vi "Main.vi"(8 "error in":errorcluster, 11 "gRPC Client in":refnum<class "gRPC Client.lvclass">) -> (0 "error out":errorcluster, 3 "gRPC Client out":refnum<class "gRPC Client.lvclass">)   [LabVIEW 2019, in "gRPC Client (template.proto).lvlib" / "gRPC Client.lvclass"]
doc: "The <b>Queued Message Handler</b> of the Worker that owns this VI."
uses:
  gRPC Client.lvclass
  C:/Program Files (x86)/National Instruments/LabVIEW 2019/vi.lib/addons/_Workers/Library/Classes/Worker/Worker.lvclass
  Initialization Data.ctl
  Response Cases.ctl
  <vilib>/addons/_Workers/Library/Case Label.ctl
  gRPC Client.lvclass/gRPC Client.ctl
  rwr_Create gRPC Client.ctl
  rwr_Create gRPC Client Reply.ctl
  rwr_Destroy gRPC Client.ctl
  rwr_Destroy gRPC Client Reply.ctl
  rqp_Msg_ToServer_1.ctl
  Generated_client/RPC Messages/w4lvgrpc_Msg_ToServer_1.ctl
  Generated_client/RPC Messages/w4lvgrpc_ToServer.ctl
  Generated_client/RPC Messages/w4lvgrpc_ToServer_payload/w4lvgrpc_ToServer_payload.lvclass
  Generated_client/RPC Messages/w4lvgrpc_ToServer_payload/w4lvgrpc_ToServer_payload.lvclass/w4lvgrpc_ToServer_payload.ctl
  rqp_Msg_ToServer_2.ctl
  Generated_client/RPC Messages/w4lvgrpc_Msg_ToServer_2.ctl
  rqp_Msg_ToServer_3.ctl
  Generated_client/RPC Messages/w4lvgrpc_Msg_ToServer_3.ctl
  rqp_Msg_ToServer_4.ctl
  Generated_client/RPC Messages/w4lvgrpc_Msg_ToServer_4.ctl
  rqp_Msg_ToServer_5.ctl
  Generated_client/RPC Messages/w4lvgrpc_Msg_ToServer_5.ctl
  rqp_Msg_ToServer_6.ctl
  Generated_client/RPC Messages/w4lvgrpc_Msg_ToServer_6.ctl
  rqp_Msg_ToServer_7.ctl
  Generated_client/RPC Messages/w4lvgrpc_Msg_ToServer_7.ctl
  rqp_Msg_ToServer_8.ctl
  Generated_client/RPC Messages/w4lvgrpc_Msg_ToServer_8.ctl
  rqp_Msg_ToServer_9.ctl
  Generated_client/RPC Messages/w4lvgrpc_Msg_ToServer_9.ctl
  Generated_client/RPC Messages/w4lvgrpc_ToClient_payload/w4lvgrpc_ToClient_payload.lvclass/w4lvgrpc_ToClient_payload.ctl
  rsp_Msg_ToClient_1.ctl
  Generated_client/RPC Messages/w4lvgrpc_Msg_ToClient_1.ctl
  rsp_Msg_ToClient_2.ctl
  Generated_client/RPC Messages/w4lvgrpc_Msg_ToClient_2.ctl
  rsp_Msg_ToClient_3.ctl
  Generated_client/RPC Messages/w4lvgrpc_Msg_ToClient_3.ctl
  rsp_Msg_ToClient_4.ctl
  Generated_client/RPC Messages/w4lvgrpc_Msg_ToClient_4.ctl
  rsp_Msg_ToClient_5.ctl
  Generated_client/RPC Messages/w4lvgrpc_Msg_ToClient_5.ctl
  rsp_Msg_ToClient_6.ctl
  Generated_client/RPC Messages/w4lvgrpc_Msg_ToClient_6.ctl
  rsp_Msg_ToClient_7.ctl
  Generated_client/RPC Messages/w4lvgrpc_Msg_ToClient_7.ctl
  rsp_Msg_ToClient_8.ctl
  Generated_client/RPC Messages/w4lvgrpc_Msg_ToClient_8.ctl
  rsp_Msg_ToClient_9.ctl
  Generated_client/RPC Messages/w4lvgrpc_Msg_ToClient_9.ctl
  <vilib>/Utility/error.llb/Error Cluster From Error Code.vi
  <vilib>/ErrorRing/Error Ring.xnode
  <vilib>/addons/_Workers/Library/Workers.lvlib
  gRPC Read/gRPC Read.lvclass
  Generated_client/Generated_client.lvlib
  Generated_client/RPC Messages/w4lvgrpc_ToClient_payload/w4lvgrpc_ToClient_payload.lvclass
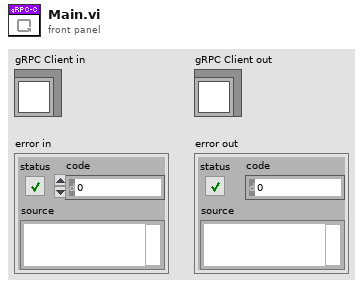
[diagram p1: front panel]
types:
  T1 = typedef "gRPC Client (template.proto).lvlib/gRPC Client.lvclass/Initialization Data.ctl" = cluster{"Response Cases":T2}
  T2 = typedef "gRPC Client (template.proto).lvlib/gRPC Client.lvclass/Response Cases.ctl" = cluster{"Connection Notify":T3, "Client Error":T3, "Msg_ToClient_1":T3, "Msg_ToClient_2":T3, "Msg_ToClient_3":T3, "Msg_ToClient_4":T3, "Msg_ToClient_5":T3, "Msg_ToClient_6":T3, "Msg_ToClient_7":T3, "Msg_ToClient_8":T3, "Msg_ToClient_9":T3}
  T3 = typedef "Workers.lvlib/Case Label.ctl" = string
  T4 = typedef "gRPC Client (template.proto).lvlib/gRPC Client.lvclass/rwr_Create gRPC Client Reply.ctl" = cluster{"Placeholder":string}
  T5 = typedef "gRPC Client (template.proto).lvlib/gRPC Client.lvclass/rwr_Create gRPC Client.ctl" = cluster{"Server Address":string, "Certificate Path":string}
  T6 = typedef "gRPC Client (template.proto).lvlib/gRPC Client.lvclass/rwr_Destroy gRPC Client Reply.ctl" = cluster{"String":string}
  T7 = typedef "gRPC Client (template.proto).lvlib/gRPC Client.lvclass/rwr_Destroy gRPC Client.ctl" = cluster{"Placeholder":string}
  T8 = typedef "Generated_client.lvlib/w4lvgrpc_ToServer.ctl" = cluster{"w4lvgrpc_ToServer_payload":refnum<class "w4lvgrpc_ToServer_payload.lvclass">}
  T9 = typedef "gRPC Client (template.proto).lvlib/gRPC Client.lvclass/rqp_Msg_ToServer_1.ctl" = cluster{"w4lvgrpc_Msg_ToServer_1":T10}
  T10 = typedef "Generated_client.lvlib/w4lvgrpc_Msg_ToServer_1.ctl" = cluster{"placeholder":string}
  T11 = typedef "gRPC Client (template.proto).lvlib/gRPC Client.lvclass/rqp_Msg_ToServer_2.ctl" = cluster{"w4lvgrpc_Msg_ToServer_2":T12}
  T12 = typedef "Generated_client.lvlib/w4lvgrpc_Msg_ToServer_2.ctl" = cluster{"placeholder":string}
  T13 = typedef "gRPC Client (template.proto).lvlib/gRPC Client.lvclass/rqp_Msg_ToServer_3.ctl" = cluster{"w4lvgrpc_Msg_ToServer_3":T14}
  T14 = typedef "Generated_client.lvlib/w4lvgrpc_Msg_ToServer_3.ctl" = cluster{"placeholder":string}
  T15 = typedef "gRPC Client (template.proto).lvlib/gRPC Client.lvclass/rqp_Msg_ToServer_4.ctl" = cluster{"w4lvgrpc_Msg_ToServer_4":T16}
  T16 = typedef "Generated_client.lvlib/w4lvgrpc_Msg_ToServer_4.ctl" = cluster{"placeholder":string}
  T17 = typedef "gRPC Client (template.proto).lvlib/gRPC Client.lvclass/rqp_Msg_ToServer_5.ctl" = cluster{"w4lvgrpc_Msg_ToServer_5":T18}
  T18 = typedef "Generated_client.lvlib/w4lvgrpc_Msg_ToServer_5.ctl" = cluster{"placeholder":string}
  T19 = typedef "gRPC Client (template.proto).lvlib/gRPC Client.lvclass/rqp_Msg_ToServer_6.ctl" = cluster{"w4lvgrpc_Msg_ToServer_6":T20}
  T20 = typedef "Generated_client.lvlib/w4lvgrpc_Msg_ToServer_6.ctl" = cluster{"placeholder":string}
  T21 = typedef "gRPC Client (template.proto).lvlib/gRPC Client.lvclass/rqp_Msg_ToServer_7.ctl" = cluster{"w4lvgrpc_Msg_ToServer_7":T22}
  T22 = typedef "Generated_client.lvlib/w4lvgrpc_Msg_ToServer_7.ctl" = cluster{"placeholder":string}
  T23 = typedef "gRPC Client (template.proto).lvlib/gRPC Client.lvclass/rqp_Msg_ToServer_8.ctl" = cluster{"w4lvgrpc_Msg_ToServer_8":T24}
  T24 = typedef "Generated_client.lvlib/w4lvgrpc_Msg_ToServer_8.ctl" = cluster{"placeholder":string}
  T25 = typedef "gRPC Client (template.proto).lvlib/gRPC Client.lvclass/rqp_Msg_ToServer_9.ctl" = cluster{"w4lvgrpc_Msg_ToServer_9":T26}
  T26 = typedef "Generated_client.lvlib/w4lvgrpc_Msg_ToServer_9.ctl" = cluster{"placeholder":string}
  T27 = typedef "gRPC Client (template.proto).lvlib/gRPC Client.lvclass/rsp_Msg_ToClient_1.ctl" = cluster{"w4lvgrpc_Msg_ToClient_1":T28}
  T28 = typedef "Generated_client.lvlib/w4lvgrpc_Msg_ToClient_1.ctl" = cluster{"placeholder":string}
  T29 = typedef "gRPC Client (template.proto).lvlib/gRPC Client.lvclass/rsp_Msg_ToClient_2.ctl" = cluster{"w4lvgrpc_Msg_ToClient_2":T30}
  T30 = typedef "Generated_client.lvlib/w4lvgrpc_Msg_ToClient_2.ctl" = cluster{"placeholder":string}
  T31 = typedef "gRPC Client (template.proto).lvlib/gRPC Client.lvclass/rsp_Msg_ToClient_3.ctl" = cluster{"w4lvgrpc_Msg_ToClient_3":T32}
  T32 = typedef "Generated_client.lvlib/w4lvgrpc_Msg_ToClient_3.ctl" = cluster{"placeholder":string}
  T33 = typedef "gRPC Client (template.proto).lvlib/gRPC Client.lvclass/rsp_Msg_ToClient_4.ctl" = cluster{"w4lvgrpc_Msg_ToClient_4":T34}
  T34 = typedef "Generated_client.lvlib/w4lvgrpc_Msg_ToClient_4.ctl" = cluster{"placeholder":string}
  T35 = typedef "gRPC Client (template.proto).lvlib/gRPC Client.lvclass/rsp_Msg_ToClient_5.ctl" = cluster{"w4lvgrpc_Msg_ToClient_5":T36}
  T36 = typedef "Generated_client.lvlib/w4lvgrpc_Msg_ToClient_5.ctl" = cluster{"placeholder":string}
  T37 = typedef "gRPC Client (template.proto).lvlib/gRPC Client.lvclass/rsp_Msg_ToClient_6.ctl" = cluster{"w4lvgrpc_Msg_ToClient_6":T38}
  T38 = typedef "Generated_client.lvlib/w4lvgrpc_Msg_ToClient_6.ctl" = cluster{"placeholder":string}
  T39 = typedef "gRPC Client (template.proto).lvlib/gRPC Client.lvclass/rsp_Msg_ToClient_7.ctl" = cluster{"w4lvgrpc_Msg_ToClient_7":T40}
  T40 = typedef "Generated_client.lvlib/w4lvgrpc_Msg_ToClient_7.ctl" = cluster{"placeholder":string}
  T41 = typedef "gRPC Client (template.proto).lvlib/gRPC Client.lvclass/rsp_Msg_ToClient_8.ctl" = cluster{"w4lvgrpc_Msg_ToClient_8":T42}
  T42 = typedef "Generated_client.lvlib/w4lvgrpc_Msg_ToClient_8.ctl" = cluster{"placeholder":string}
  T43 = typedef "gRPC Client (template.proto).lvlib/gRPC Client.lvclass/rsp_Msg_ToClient_9.ctl" = cluster{"w4lvgrpc_Msg_ToClient_9":T44}
  T44 = typedef "Generated_client.lvlib/w4lvgrpc_Msg_ToClient_9.ctl" = cluster{"placeholder":string}
  T45 = typedef "grpc-lvsupport-release.lvlib/grpcId.ctl" = u64
  T46 = typedef "gRPC Client (template.proto).lvlib/gRPC Read.lvclass/rsp_Receive Incoming gRPC Data.ctl" = refnum<class "w4lvgrpc_ToClient_payload.lvclass">
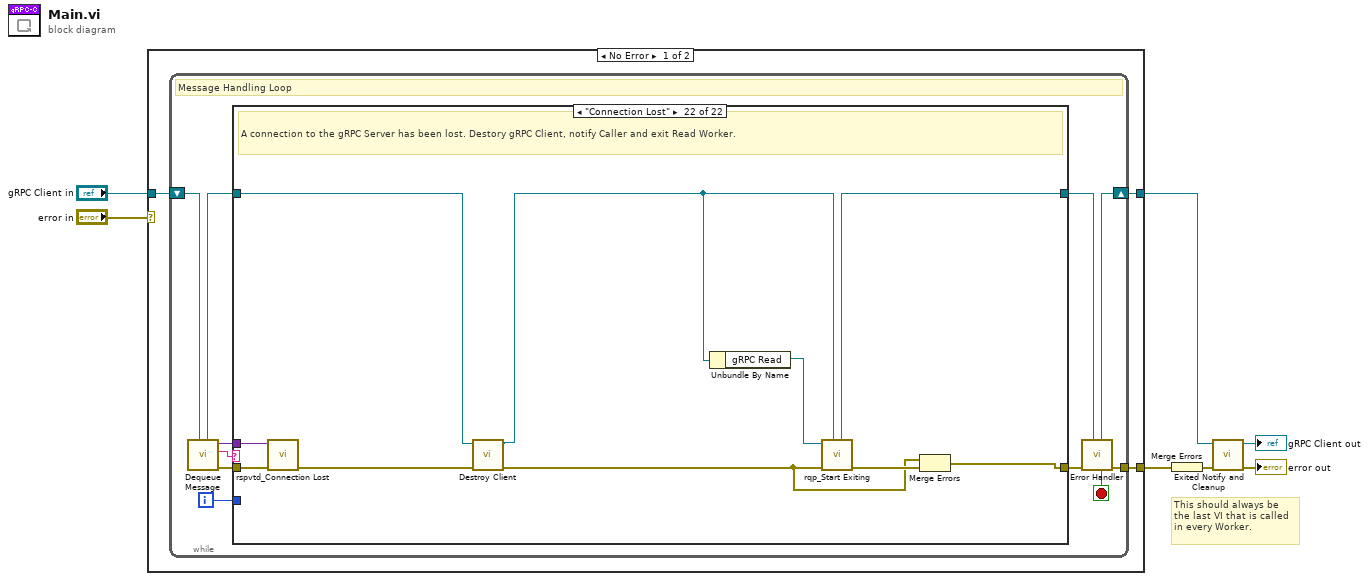
[diagram p0: block diagram]
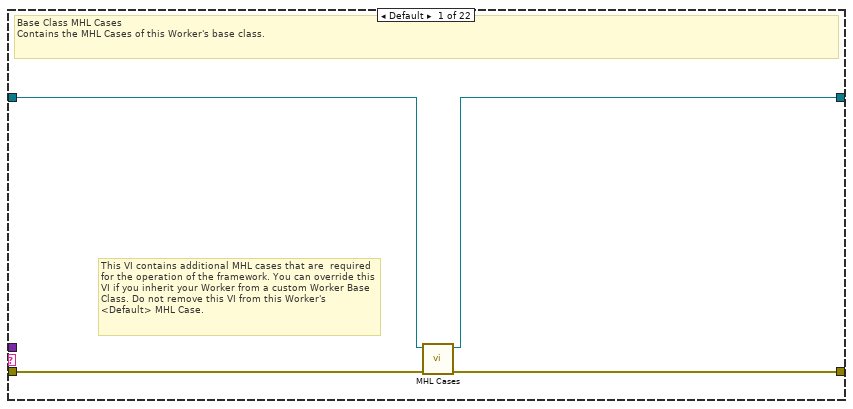
[diagram p2: hidden frame]
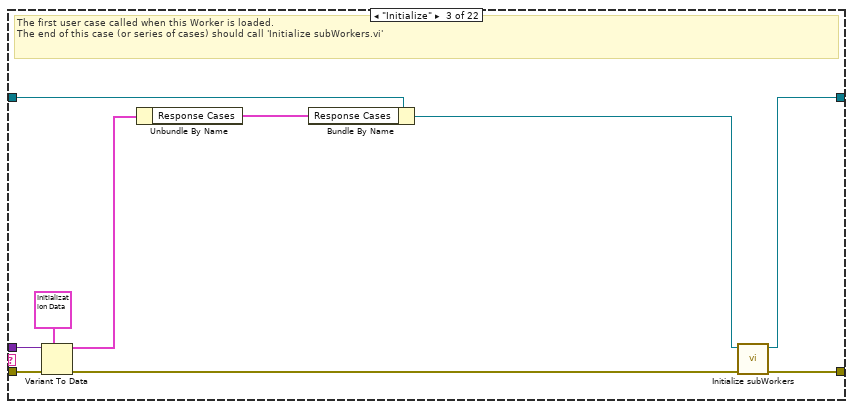
[diagram p4: hidden frame]
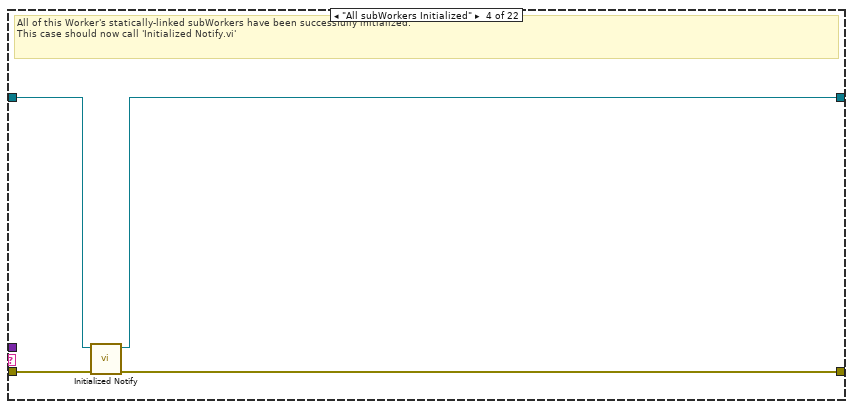
[diagram p5: hidden frame]
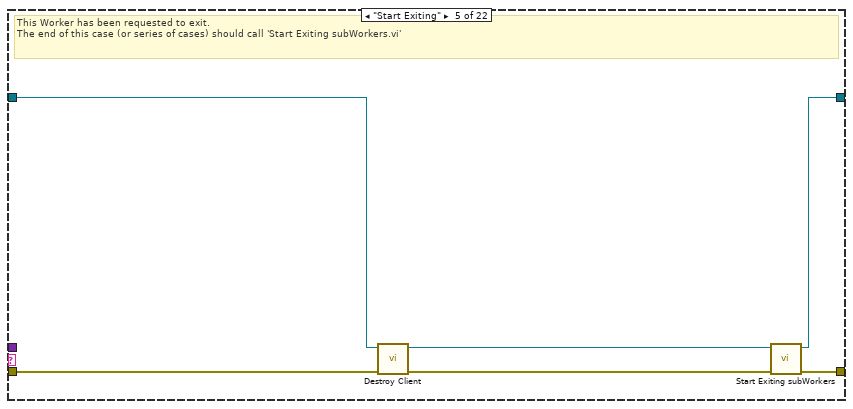
[diagram p6: hidden frame]
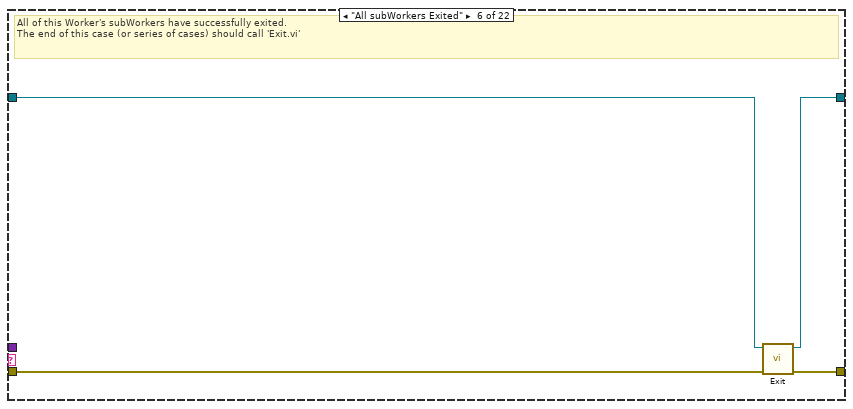
[diagram p7: hidden frame]
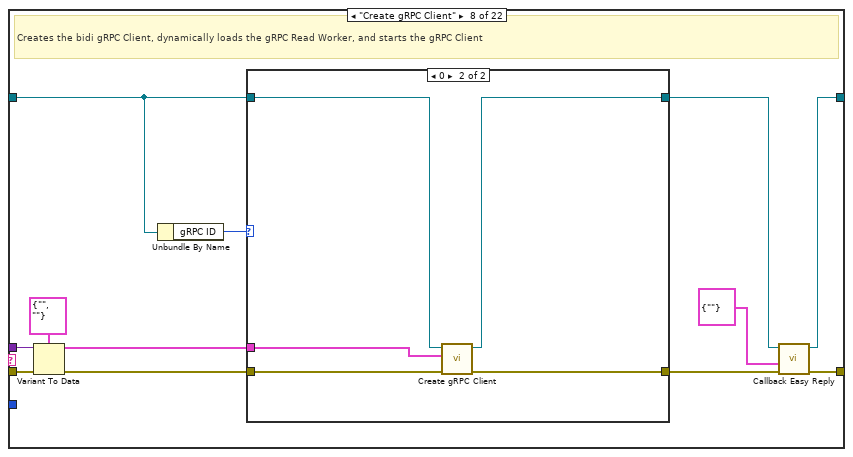
[diagram p9: hidden frame]
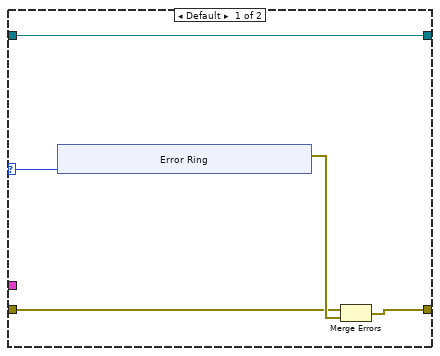
[diagram p10: hidden frame]
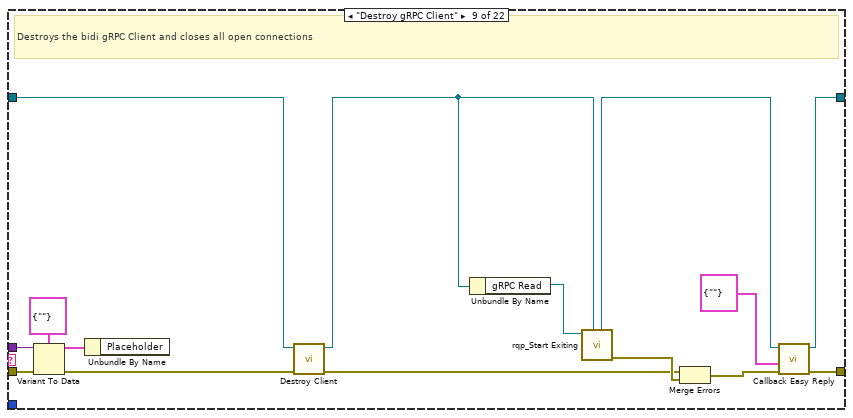
[diagram p11: hidden frame]
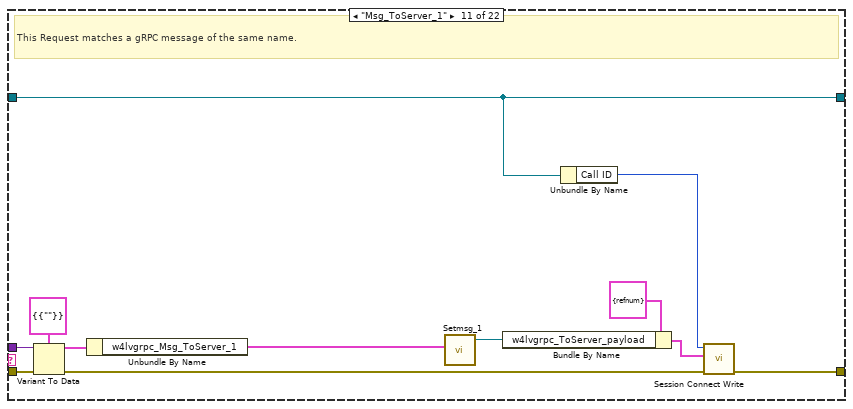
[diagram p13: hidden frame]
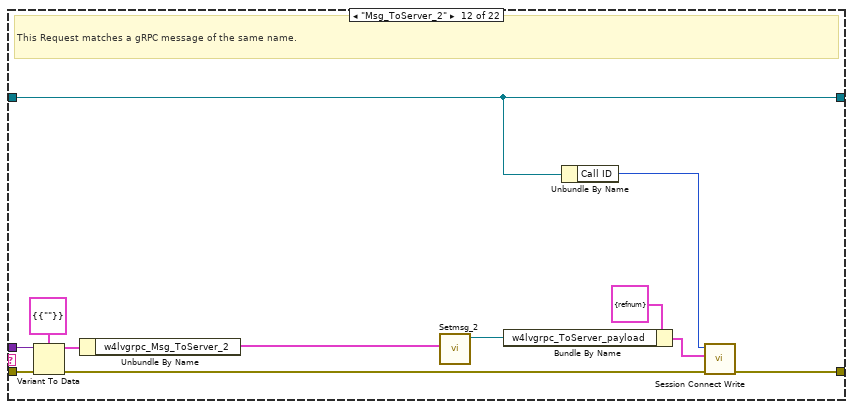
[diagram p14: hidden frame]
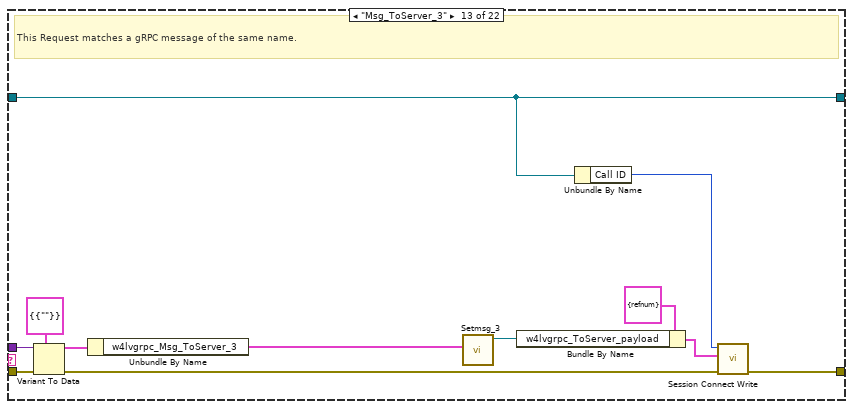
[diagram p15: hidden frame]
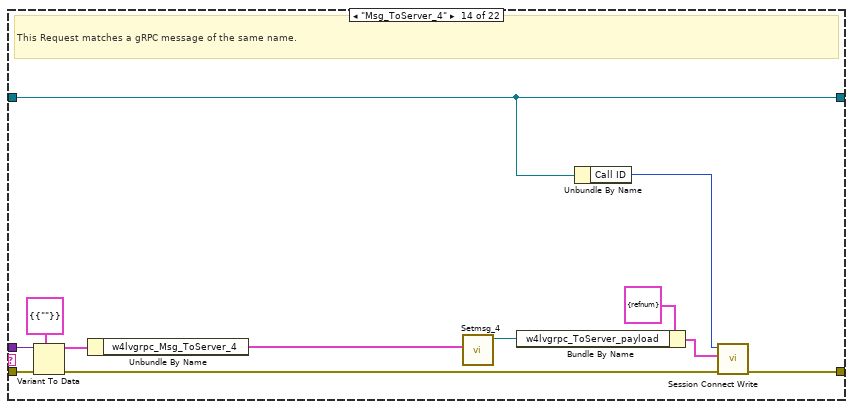
[diagram p16: hidden frame]
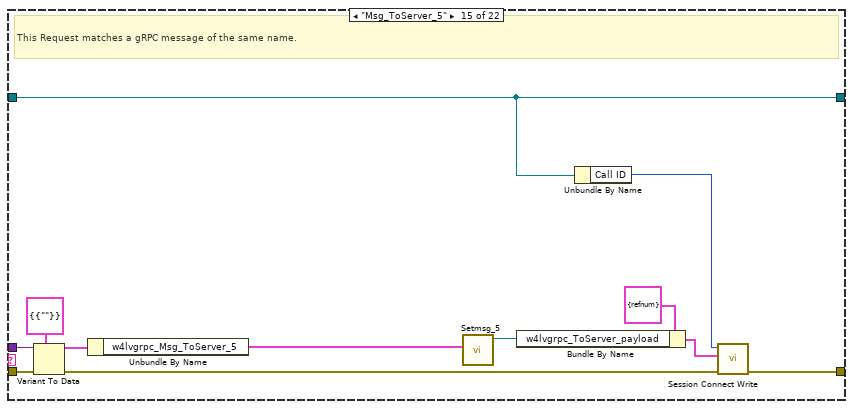
[diagram p17: hidden frame]
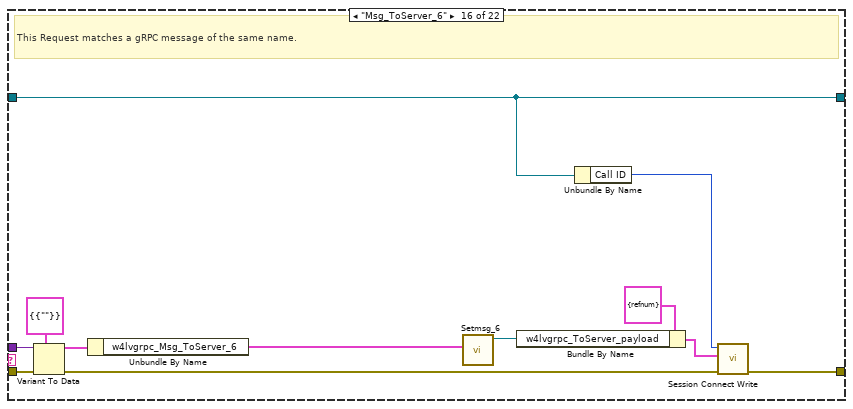
[diagram p18: hidden frame]
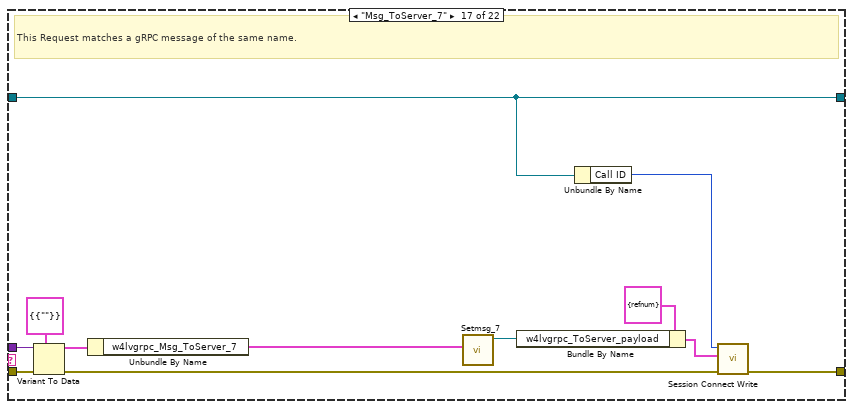
[diagram p19: hidden frame]
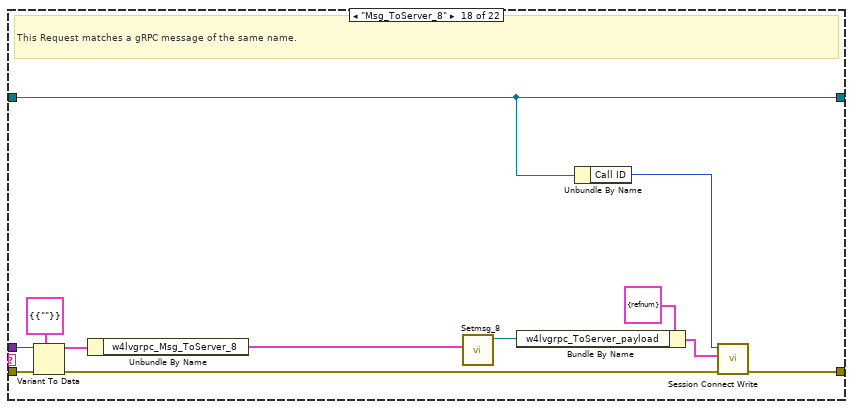
[diagram p20: hidden frame]
diagram:
  # "This should always be the last VI that is called in every Worker."
  n1 = case shown="No Error" "error in" {
    tunnel: "gRPC Client in" -> [w10 w324]
    tunnel: [w8 w325] -> w5
    tunnel: [w9 w323] -> w6
    selector: "error in" -> [_ w326]
    frame No Error {
      n2 = while {
        shift-right: [w19] -> w9
        shift-left: w10 -> [w21]
        tunnel: [w20] -> w8
        i -> [w12]
        stop <- w13 stop-if-true
        # "Message Handling Loop"
        n3 = call-dynamic "Dequeue Message.vi"("Worker"=w21) -> ("error out"=w18:errorcluster, "Case out"=w14:string, "Data out"=w11:variant, "Worker out"=w16:refnum<class "gRPC Client.lvclass">)  [unwired: 6 in, 1 out]
        n4 = case "Worker MHL Case Structure (DO NOT CHANGE LABEL NAME)" shown="\"Connection Lost\"" w14 {
          tunnel: w18 -> [w25 w26 w35 w39 w45 w51 w53 w65 w97 w99 w111 w123 w135 w147 w159 w171 w183 w195 w207 w209 w215 w321]
          tunnel: [w24 w26 w37 w38 w47 w50 w53 w62 w93 w99 w103 w112 w129 w141 w153 w165 w177 w189 w201 w209 w219 w315] -> w17
          tunnel: w16 -> [w23 w27 w34 w41 w42 w49 w52 w54 w89 w98 w102 w116 w131 w143 w155 w167 w179 w191 w203 w208 w218 w319]
          tunnel: [w22 w27 w36 w40 w46 w48 w52 w61 w92 w98 w102 w116 w131 w143 w155 w167 w179 w191 w203 w208 w217 w313] -> w15
          tunnel: w12 -> [_ _ _ _ _ _ _ _ _ _ _ _ _ _ _ _ _ _ _ _ _ _]
          tunnel: w11 -> [_ _ w32 _ _ _ _ w63 w95 _ w109 w121 w133 w145 w157 w169 w181 w193 w205 _ w216 w322]
          frame Default {
            # "This VI contains additional MHL cases that are  required for the operation of the framework. You can override this VI if you inherit your Worker from a custom Worker Base Class. Do not remove this VI from this Worker's <Default> MHL Case."
            # "Base Class MHL Cases\nContains the MHL Cases of this Worker's base class."
            n5 = call-dynamic "MHL Cases.vi"("error in"=w25, "Worker in"=w23) -> ("error out"=w24:errorcluster, "Worker out"=w22:refnum<class "gRPC Client.lvclass">)  [unwired: 8 in]
          }
          frame "------------ FRAMEWORK CASES -----------" {
            # "Start of Workers Framework Cases"
          }
          frame "Initialize" {
            # "The first user case called when this Worker is loaded.\nThe end of this case (or series of cases) should call 'Initialize subWorkers.vi'"
            n6 = Variant To Data(error in=w35, type=T1 {"Response Cases"={"Connection Notify"="", "Client Error"="", "Msg_ToClient_1"="", "Msg_ToClient_2"="", "Msg_ToClient_3"="", "Msg_ToClient_4"="", "Msg_ToClient_5"="", "Msg_ToClient_6"="", "Msg_ToClient_7"="", "Msg_ToClient_8"="", "Msg_ToClient_9"=""}} ("Initialization Data"), Variant=w32) -> (data=w31:T1, error out=w33:errorcluster)
            n7 = Unbundle By Name(w31) -> ("Response Cases"=w30:T2)
            n8 = Bundle By Name(cluster=w34, "Response Cases"=w30) -> (w28:refnum<class "gRPC Client.lvclass">)
            n9 = call-dynamic "Initialize subWorkers.vi"("error in"=w33, "Worker"=w28) -> ("error out"=w37:errorcluster, "dup Worker out"=w36:refnum<class "gRPC Client.lvclass">)  [unwired: 8 in]
          }
          frame "All subWorkers Initialized" {
            # "All of this Worker's statically-linked subWorkers have been successfully initialized.\nThis case should now call 'Initialized Notify.vi'"
            n10 = call-dynamic "Initialized Notify.vi"("error in"=w39, "Worker"=w41) -> ("error out"=w38:errorcluster, "dup Worker out"=w40:refnum<class "gRPC Client.lvclass">)  [unwired: 8 in]
          }
          frame "Start Exiting" {
            # "This Worker has been requested to exit. \nThe end of this case (or series of cases) should call 'Start Exiting subWorkers.vi'"
            n11 = call "Destroy Client.vi"("error in (no error)"=w45, "gRPC Client in"=w42) -> ("error out"=w44:errorcluster, "gRPC Client out"=w43:refnum<class "gRPC Client.lvclass">)  [unwired: 8 in]
            n12 = call-dynamic "Start Exiting subWorkers.vi"("error_in"=w44, "Worker"=w43) -> ("error out"=w47:errorcluster, "dup Worker out"=w46:refnum<class "gRPC Client.lvclass">)  [unwired: 8 in]
          }
          frame "All subWorkers Exited" {
            # "All of this Worker's subWorkers have successfully exited. \nThe end of this case (or series of cases) should call 'Exit.vi'"
            n13 = call-dynamic "Exit.vi"("error_in"=w51, "Worker"=w49) -> ("error out"=w50:errorcluster, "dup Worker out"=w48:refnum<class "gRPC Client.lvclass">)  [unwired: 8 in]
          }
          frame "------------- PUBLIC API CASES -------------" {
            # "Start of Workers Public API Cases"
          }
          frame "Create gRPC Client" {
            # "Creates the bidi gRPC Client, dynamically loads the gRPC Read Worker, and starts the gRPC Client"
            n14 = Variant To Data(error in=w65, type=T5 {"Server Address"="", "Certificate Path"=""} ("Data"), Variant=w63) -> (data=w58:T5, error out=w59:errorcluster)
            n15 = Unbundle By Name(w54) -> ("gRPC ID"=w55:T45)
            n16 = case shown="0" w55 {
              selector: w55 -> [w66 _]
              tunnel: w54 -> [w70 w82]
              tunnel: w59 -> [w67 w81]
              tunnel: w58 -> [_ w80]
              tunnel: [w69 w78] -> w57
              tunnel: [w70 w79] -> w56
              frame Default {
                n17 = xnode "Error Ring"("parameter 0"=w66) -> ("error out"=w68:errorcluster)
                n18 = Merge Errors(w67, w68) -> (w69:errorcluster)
              }
              frame 0 {
                n19 = call "Create gRPC Client.vi"("error in (no error)"=w81, "Data"=w80, "gRPC Client in"=w82) -> ("error out"=w78:errorcluster, "gRPC Client out"=w79:refnum<class "gRPC Client.lvclass">)  [unwired: 7 in]
              }
            }
            n20 = call-dynamic "Callback Easy Reply.vi"("error in"=w57, "Data"=T4 {"Placeholder"=""} ("Reply Data"), "Worker"=w56) -> ("error out"=w62:errorcluster, "dup Worker out"=w61:refnum<class "gRPC Client.lvclass">)  [unwired: 7 in]
          }
          frame "Destroy gRPC Client" {
            # "Destroys the bidi gRPC Client and closes all open connections"
            n21 = Variant To Data(error in=w97, type=T7 {"Placeholder"=""} ("Data"), Variant=w95) -> (data=w94:T7, error out=w90:errorcluster)
            n22 = Unbundle By Name(w94) -> ()  [unwired: 1 out]
            n23 = call "Destroy Client.vi"("error in (no error)"=w90, "gRPC Client in"=w89) -> ("error out"=w83:errorcluster, "gRPC Client out"=w86:refnum<class "gRPC Client.lvclass">)  [unwired: 8 in]
            n24 = Unbundle By Name(w86) -> ("gRPC Read"=w85:refnum<class "gRPC Read.lvclass">)
            n25 = call "rqp_Start Exiting.vi"("Caller in"=w86, "gRPC Read in"=w85) -> ("error out"=w87:errorcluster, "dup Caller out"=w88:refnum<class "gRPC Client.lvclass">)  [unwired: 7 in, 1 out]
            n26 = Merge Errors(w83, w87) -> (w84:errorcluster)
            n27 = call-dynamic "Callback Easy Reply.vi"("error in"=w84, "Data"=T6 {"String"=""} ("Reply Data"), "Worker"=w88) -> ("error out"=w93:errorcluster, "dup Worker out"=w92:refnum<class "gRPC Client.lvclass">)  [unwired: 7 in]
          }
          frame "~~~~~~~~ gRPC Messages ~~~~~~~~~~ " {
          }
          frame "Msg_ToServer_1" {
            # "This Request matches a gRPC message of the same name."
            n28 = Variant To Data(error in=w111, type=T9 {"w4lvgrpc_Msg_ToServer_1"={"placeholder"=""}} ("Data"), Variant=w109) -> (data=w108:T9, error out=w104:errorcluster)
            n29 = Unbundle By Name(w108) -> ("w4lvgrpc_Msg_ToServer_1"=w100:T10)
            n30 = call "Setmsg_1.vi"("Set_Val"=w100) -> ("OneOfTemplate out"=w101:refnum<class "w4lvgrpc_ToServer_payload.lvclass">)  [unwired: 9 in, 1 out]
            n31 = Bundle By Name(cluster=T8 {"w4lvgrpc_ToServer_payload"=refnum} ("Message Data"), "w4lvgrpc_ToServer_payload"=w101) -> (w105:T8)
            n32 = Unbundle By Name(w102) -> ("Call ID"=w107:T45)
            n33 = call "Session Connect Write.vi"("error in"=w104, "Request Data"=w105, "Call ID in"=w107) -> ("error out"=w103:errorcluster)  [unwired: 6 in, 2 out]
          }
          frame "Msg_ToServer_2" {
            # "This Request matches a gRPC message of the same name."
            n34 = Variant To Data(error in=w123, type=T11 {"w4lvgrpc_Msg_ToServer_2"={"placeholder"=""}} ("Data"), Variant=w121) -> (data=w120:T11, error out=w113:errorcluster)
            n35 = Unbundle By Name(w120) -> ("w4lvgrpc_Msg_ToServer_2"=w114:T12)
            n36 = call "Setmsg_2.vi"("Set_Val"=w114) -> ("OneOfTemplate out"=w115:refnum<class "w4lvgrpc_ToServer_payload.lvclass">)  [unwired: 9 in, 1 out]
            n37 = Bundle By Name(cluster=T8 {"w4lvgrpc_ToServer_payload"=refnum} ("Message Data"), "w4lvgrpc_ToServer_payload"=w115) -> (w117:T8)
            n38 = Unbundle By Name(w116) -> ("Call ID"=w119:T45)
            n39 = call "Session Connect Write.vi"("error in"=w113, "Request Data"=w117, "Call ID in"=w119) -> ("error out"=w112:errorcluster)  [unwired: 6 in, 2 out]
          }
          frame "Msg_ToServer_3" {
            # "This Request matches a gRPC message of the same name."
            n40 = Variant To Data(error in=w135, type=T13 {"w4lvgrpc_Msg_ToServer_3"={"placeholder"=""}} ("Data"), Variant=w133) -> (data=w132:T13, error out=w128:errorcluster)
            n41 = Unbundle By Name(w132) -> ("w4lvgrpc_Msg_ToServer_3"=w125:T14)
            n42 = call "Setmsg_3.vi"("Set_Val"=w125) -> ("OneOfTemplate out"=w124:refnum<class "w4lvgrpc_ToServer_payload.lvclass">)  [unwired: 9 in, 1 out]
            n43 = Bundle By Name(cluster=T8 {"w4lvgrpc_ToServer_payload"=refnum} ("Message Data"), "w4lvgrpc_ToServer_payload"=w124) -> (w126:T8)
            n44 = Unbundle By Name(w131) -> ("Call ID"=w130:T45)
            n45 = call "Session Connect Write.vi"("error in"=w128, "Request Data"=w126, "Call ID in"=w130) -> ("error out"=w129:errorcluster)  [unwired: 6 in, 2 out]
          }
          frame "Msg_ToServer_4" {
            # "This Request matches a gRPC message of the same name."
            n46 = Variant To Data(error in=w147, type=T15 {"w4lvgrpc_Msg_ToServer_4"={"placeholder"=""}} ("Data"), Variant=w145) -> (data=w144:T15, error out=w140:errorcluster)
            n47 = Unbundle By Name(w144) -> ("w4lvgrpc_Msg_ToServer_4"=w136:T16)
            n48 = call "Setmsg_4.vi"("Set_Val"=w136) -> ("OneOfTemplate out"=w137:refnum<class "w4lvgrpc_ToServer_payload.lvclass">)  [unwired: 9 in, 1 out]
            n49 = Bundle By Name(cluster=T8 {"w4lvgrpc_ToServer_payload"=refnum} ("Message Data"), "w4lvgrpc_ToServer_payload"=w137) -> (w138:T8)
            n50 = Unbundle By Name(w143) -> ("Call ID"=w142:T45)
            n51 = call "Session Connect Write.vi"("error in"=w140, "Request Data"=w138, "Call ID in"=w142) -> ("error out"=w141:errorcluster)  [unwired: 6 in, 2 out]
          }
          frame "Msg_ToServer_5" {
            # "This Request matches a gRPC message of the same name."
            n52 = Variant To Data(error in=w159, type=T17 {"w4lvgrpc_Msg_ToServer_5"={"placeholder"=""}} ("Data"), Variant=w157) -> (data=w156:T17, error out=w152:errorcluster)
            n53 = Unbundle By Name(w156) -> ("w4lvgrpc_Msg_ToServer_5"=w148:T18)
            n54 = call "Setmsg_5.vi"("Set_Val"=w148) -> ("OneOfTemplate out"=w149:refnum<class "w4lvgrpc_ToServer_payload.lvclass">)  [unwired: 9 in, 1 out]
            n55 = Bundle By Name(cluster=T8 {"w4lvgrpc_ToServer_payload"=refnum} ("Message Data"), "w4lvgrpc_ToServer_payload"=w149) -> (w150:T8)
            n56 = Unbundle By Name(w155) -> ("Call ID"=w154:T45)
            n57 = call "Session Connect Write.vi"("error in"=w152, "Request Data"=w150, "Call ID in"=w154) -> ("error out"=w153:errorcluster)  [unwired: 6 in, 2 out]
          }
          frame "Msg_ToServer_6" {
            # "This Request matches a gRPC message of the same name."
            n58 = Variant To Data(error in=w171, type=T19 {"w4lvgrpc_Msg_ToServer_6"={"placeholder"=""}} ("Data"), Variant=w169) -> (data=w168:T19, error out=w164:errorcluster)
            n59 = Unbundle By Name(w168) -> ("w4lvgrpc_Msg_ToServer_6"=w160:T20)
            n60 = call "Setmsg_6.vi"("Set_Val"=w160) -> ("OneOfTemplate out"=w161:refnum<class "w4lvgrpc_ToServer_payload.lvclass">)  [unwired: 9 in, 1 out]
            n61 = Bundle By Name(cluster=T8 {"w4lvgrpc_ToServer_payload"=refnum} ("Message Data"), "w4lvgrpc_ToServer_payload"=w161) -> (w162:T8)
            n62 = Unbundle By Name(w167) -> ("Call ID"=w166:T45)
            n63 = call "Session Connect Write.vi"("error in"=w164, "Request Data"=w162, "Call ID in"=w166) -> ("error out"=w165:errorcluster)  [unwired: 6 in, 2 out]
          }
          frame "Msg_ToServer_7" {
            # "This Request matches a gRPC message of the same name."
            n64 = Variant To Data(error in=w183, type=T21 {"w4lvgrpc_Msg_ToServer_7"={"placeholder"=""}} ("Data"), Variant=w181) -> (data=w180:T21, error out=w176:errorcluster)
            n65 = Unbundle By Name(w180) -> ("w4lvgrpc_Msg_ToServer_7"=w172:T22)
            n66 = call "Setmsg_7.vi"("Set_Val"=w172) -> ("OneOfTemplate out"=w173:refnum<class "w4lvgrpc_ToServer_payload.lvclass">)  [unwired: 9 in, 1 out]
            n67 = Bundle By Name(cluster=T8 {"w4lvgrpc_ToServer_payload"=refnum} ("Message Data"), "w4lvgrpc_ToServer_payload"=w173) -> (w174:T8)
            n68 = Unbundle By Name(w179) -> ("Call ID"=w178:T45)
            n69 = call "Session Connect Write.vi"("error in"=w176, "Request Data"=w174, "Call ID in"=w178) -> ("error out"=w177:errorcluster)  [unwired: 6 in, 2 out]
          }
          frame "Msg_ToServer_8" {
            # "This Request matches a gRPC message of the same name."
            n70 = Variant To Data(error in=w195, type=T23 {"w4lvgrpc_Msg_ToServer_8"={"placeholder"=""}} ("Data"), Variant=w193) -> (data=w192:T23, error out=w188:errorcluster)
            n71 = Unbundle By Name(w192) -> ("w4lvgrpc_Msg_ToServer_8"=w184:T24)
            n72 = call "Setmsg_8.vi"("Set_Val"=w184) -> ("OneOfTemplate out"=w185:refnum<class "w4lvgrpc_ToServer_payload.lvclass">)  [unwired: 9 in, 1 out]
            n73 = Bundle By Name(cluster=T8 {"w4lvgrpc_ToServer_payload"=refnum} ("Message Data"), "w4lvgrpc_ToServer_payload"=w185) -> (w186:T8)
            n74 = Unbundle By Name(w191) -> ("Call ID"=w190:T45)
            n75 = call "Session Connect Write.vi"("error in"=w188, "Request Data"=w186, "Call ID in"=w190) -> ("error out"=w189:errorcluster)  [unwired: 6 in, 2 out]
          }
          frame "Msg_ToServer_9" {
            # "This Request matches a gRPC message of the same name."
            n76 = Variant To Data(error in=w207, type=T25 {"w4lvgrpc_Msg_ToServer_9"={"placeholder"=""}} ("Data"), Variant=w205) -> (data=w204:T25, error out=w200:errorcluster)
            n77 = Unbundle By Name(w204) -> ("w4lvgrpc_Msg_ToServer_9"=w196:T26)
            n78 = call "Setmsg_9.vi"("Set_Val"=w196) -> ("OneOfTemplate out"=w197:refnum<class "w4lvgrpc_ToServer_payload.lvclass">)  [unwired: 9 in, 1 out]
            n79 = Bundle By Name(cluster=T8 {"w4lvgrpc_ToServer_payload"=refnum} ("Message Data"), "w4lvgrpc_ToServer_payload"=w197) -> (w198:T8)
            n80 = Unbundle By Name(w203) -> ("Call ID"=w202:T45)
            n81 = call "Session Connect Write.vi"("error in"=w200, "Request Data"=w198, "Call ID in"=w202) -> ("error out"=w201:errorcluster)  [unwired: 6 in, 2 out]
          }
          frame "------------- RESPONSE CASES --------------" {
            # "Start of Workers Response Cases"
          }
          frame "Receive Incoming gRPC Data" {
            # "*** IMPORTANT ***\n\nCase Selector must match index of gRPC ProtoBuf ToServer oneof payload"
            # "This case receives incoming data from a gRPC Server, and then delegates the data to the associated Public Response"
            n82 = call "rspvtd_Receive Incoming gRPC Data.vi"("error in"=w215, "Data in"=w216) -> ("error out"=w213:errorcluster, "Data out"=w214:T46)  [unwired: 8 in]
            n83 = call "GetActiveFieldIndex.vi"("error in (no error)"=w213, "OneOfTemplate in"=w214) -> ("error out"=w210:errorcluster, "Active Field Index"=w211:i32, "OneOfTemplate out"=w212:T46)  [unwired: 7 in]
            n84 = case shown="1" w211 {
              selector: w211 -> [w220 _ _ _ _ _ _ _ _ _]
              tunnel: w210 -> [w221 w236 w245 w254 w263 w272 w281 w290 w299 w308]
              tunnel: [w222 w240 w249 w258 w267 w276 w285 w294 w303 w312] -> w219
              tunnel: w218 -> [w224 w239 w248 w257 w266 w275 w284 w293 w302 w311]
              tunnel: [w224 w238 w247 w256 w265 w274 w283 w292 w301 w310] -> w217
              tunnel: w212 -> [_ w237 w246 w255 w264 w273 w282 w291 w300 w309]
              frame Default {
                n85 = xnode "Error Ring"("parameter 0"=w220) -> ("error out"=w223:errorcluster)
                n86 = Merge Errors(w221, w223) -> (w222:errorcluster)
              }
              frame 1 {
                n87 = call "Getmsg_1.vi"("error in (no error)"=w236, "OneOfTemplate in"=w237) -> ("error out"=w235:errorcluster, "Get_Val"=w232:T28)  [unwired: 7 in, 1 out]
                n88 = Bundle By Name(cluster=T27 {"w4lvgrpc_Msg_ToClient_1"={"placeholder"=""}} ("Data in"), "w4lvgrpc_Msg_ToClient_1"=w232) -> (w233:T27)
                n89 = call "rsp_Msg_ToClient_1.vi"("error in"=w235, "Data in"=w233, "gRPC Client in"=w239) -> ("error out"=w240:errorcluster, "dup gRPC Client out"=w238:refnum<class "gRPC Client.lvclass">)  [unwired: 7 in]
              }
              frame 2 {
                n90 = call "Getmsg_2.vi"("error in (no error)"=w245, "OneOfTemplate in"=w246) -> ("error out"=w244:errorcluster, "Get_Val"=w241:T30)  [unwired: 7 in, 1 out]
                n91 = Bundle By Name(cluster=T29 {"w4lvgrpc_Msg_ToClient_2"={"placeholder"=""}} ("Data in"), "w4lvgrpc_Msg_ToClient_2"=w241) -> (w242:T29)
                n92 = call "rsp_Msg_ToClient_2.vi"("error in"=w244, "Data in"=w242, "gRPC Client in"=w248) -> ("error out"=w249:errorcluster, "dup gRPC Client out"=w247:refnum<class "gRPC Client.lvclass">)  [unwired: 7 in]
              }
              frame 3 {
                n93 = call "Getmsg_3.vi"("error in (no error)"=w254, "OneOfTemplate in"=w255) -> ("error out"=w253:errorcluster, "Get_Val"=w250:T32)  [unwired: 7 in, 1 out]
                n94 = Bundle By Name(cluster=T31 {"w4lvgrpc_Msg_ToClient_3"={"placeholder"=""}} ("Data in"), "w4lvgrpc_Msg_ToClient_3"=w250) -> (w251:T31)
                n95 = call "rsp_Msg_ToClient_3.vi"("error in"=w253, "Data in"=w251, "gRPC Client in"=w257) -> ("error out"=w258:errorcluster, "dup gRPC Client out"=w256:refnum<class "gRPC Client.lvclass">)  [unwired: 7 in]
              }
              frame 4 {
                n96 = call "Getmsg_4.vi"("error in (no error)"=w263, "OneOfTemplate in"=w264) -> ("error out"=w262:errorcluster, "Get_Val"=w259:T34)  [unwired: 7 in, 1 out]
                n97 = Bundle By Name(cluster=T33 {"w4lvgrpc_Msg_ToClient_4"={"placeholder"=""}} ("Data in"), "w4lvgrpc_Msg_ToClient_4"=w259) -> (w260:T33)
                n98 = call "rsp_Msg_ToClient_4.vi"("error in"=w262, "Data in"=w260, "gRPC Client in"=w266) -> ("error out"=w267:errorcluster, "dup gRPC Client out"=w265:refnum<class "gRPC Client.lvclass">)  [unwired: 7 in]
              }
              frame 5 {
                n99 = call "Getmsg_5.vi"("error in (no error)"=w272, "OneOfTemplate in"=w273) -> ("error out"=w271:errorcluster, "Get_Val"=w268:T36)  [unwired: 7 in, 1 out]
                n100 = Bundle By Name(cluster=T35 {"w4lvgrpc_Msg_ToClient_5"={"placeholder"=""}} ("Data in"), "w4lvgrpc_Msg_ToClient_5"=w268) -> (w269:T35)
                n101 = call "rsp_Msg_ToClient_5.vi"("error in"=w271, "Data in"=w269, "gRPC Client in"=w275) -> ("error out"=w276:errorcluster, "dup gRPC Client out"=w274:refnum<class "gRPC Client.lvclass">)  [unwired: 7 in]
              }
              frame 6 {
                n102 = call "Getmsg_6.vi"("error in (no error)"=w281, "OneOfTemplate in"=w282) -> ("error out"=w280:errorcluster, "Get_Val"=w277:T38)  [unwired: 7 in, 1 out]
                n103 = Bundle By Name(cluster=T37 {"w4lvgrpc_Msg_ToClient_6"={"placeholder"=""}} ("Data in"), "w4lvgrpc_Msg_ToClient_6"=w277) -> (w278:T37)
                n104 = call "rsp_Msg_ToClient_6.vi"("error in"=w280, "Data in"=w278, "gRPC Client in"=w284) -> ("error out"=w285:errorcluster, "dup gRPC Client out"=w283:refnum<class "gRPC Client.lvclass">)  [unwired: 7 in]
              }
              frame 7 {
                n105 = call "Getmsg_7.vi"("error in (no error)"=w290, "OneOfTemplate in"=w291) -> ("error out"=w289:errorcluster, "Get_Val"=w286:T40)  [unwired: 7 in, 1 out]
                n106 = Bundle By Name(cluster=T39 {"w4lvgrpc_Msg_ToClient_7"={"placeholder"=""}} ("Data in"), "w4lvgrpc_Msg_ToClient_7"=w286) -> (w287:T39)
                n107 = call "rsp_Msg_ToClient_7.vi"("error in"=w289, "Data in"=w287, "gRPC Client in"=w293) -> ("error out"=w294:errorcluster, "dup gRPC Client out"=w292:refnum<class "gRPC Client.lvclass">)  [unwired: 7 in]
              }
              frame 8 {
                n108 = call "Getmsg_8.vi"("error in (no error)"=w299, "OneOfTemplate in"=w300) -> ("error out"=w298:errorcluster, "Get_Val"=w295:T42)  [unwired: 7 in, 1 out]
                n109 = Bundle By Name(cluster=T41 {"w4lvgrpc_Msg_ToClient_8"={"placeholder"=""}} ("Data in"), "w4lvgrpc_Msg_ToClient_8"=w295) -> (w296:T41)
                n110 = call "rsp_Msg_ToClient_8.vi"("error in"=w298, "Data in"=w296, "gRPC Client in"=w302) -> ("error out"=w303:errorcluster, "dup gRPC Client out"=w301:refnum<class "gRPC Client.lvclass">)  [unwired: 7 in]
              }
              frame 9 {
                n111 = call "Getmsg_9.vi"("error in (no error)"=w308, "OneOfTemplate in"=w309) -> ("error out"=w307:errorcluster, "Get_Val"=w304:T44)  [unwired: 7 in, 1 out]
                n112 = Bundle By Name(cluster=T43 {"w4lvgrpc_Msg_ToClient_9"={"placeholder"=""}} ("Data in"), "w4lvgrpc_Msg_ToClient_9"=w304) -> (w305:T43)
                n113 = call "rsp_Msg_ToClient_9.vi"("error in"=w307, "Data in"=w305, "gRPC Client in"=w311) -> ("error out"=w312:errorcluster, "dup gRPC Client out"=w310:refnum<class "gRPC Client.lvclass">)  [unwired: 7 in]
              }
            }
          }
          frame "Connection Lost" {
            # "A connection to the gRPC Server has been lost. Destory gRPC Client, notify Caller and exit Read Worker."
            n114 = call "rspvtd_Connection Lost.vi"("error in"=w321, "Data in"=w322) -> ("error out"=w320:errorcluster)  [unwired: 8 in, 1 out]
            n115 = call "Destroy Client.vi"("error in (no error)"=w320, "gRPC Client in"=w319) -> ("error out"=w316:errorcluster, "gRPC Client out"=w314:refnum<class "gRPC Client.lvclass">)  [unwired: 8 in]
            n116 = Unbundle By Name(w314) -> ("gRPC Read"=w317:refnum<class "gRPC Read.lvclass">)
            n117 = call "rqp_Start Exiting.vi"("Caller in"=w314, "error in"=w316, "gRPC Read in"=w317) -> ("error out"=w318:errorcluster, "dup Caller out"=w313:refnum<class "gRPC Client.lvclass">)  [unwired: 6 in, 1 out]
            n118 = Merge Errors(w316, w318) -> (w315:errorcluster)
          }
        }
        n119 = call-dynamic "Error Handler.vi"("gRPC Client"=w15, "error_in"=w17) -> ("error out"=w20:errorcluster, "Stop Loop"=w13:bool, "gRPC Client out"=w19:refnum<class "gRPC Client.lvclass">)  [unwired: 7 in]
      }
    }
    frame Error {
      n120 = call-dynamic "Error Handler.vi"("gRPC Client"=w324, "error_in"=w326) -> ("error out"=w325:errorcluster, "gRPC Client out"=w323:refnum<class "gRPC Client.lvclass">)  [unwired: 7 in, 1 out]
    }
  }
  n121 = Merge Errors(w5) -> (w7:errorcluster)
  n122 = call-dynamic "Exited Notify and Cleanup.vi"("error_in"=w7, "Worker"=w6) -> ("error out"=→"error out":errorcluster, "dup Worker out"=→"gRPC Client out":refnum<class "gRPC Client.lvclass">)  [unwired: 8 in]
